vi "灯值调整写入.vi"(8 "error in (no error)":errorcluster, 11 "写入值":cluster{"波长":u16, "ADC":u16, "目标值":u16}={"波长"=365, "ADC"=0, "目标值"=0} {"波长" items=["365"=365, "520"=520, "660"=660]}) -> (0 "error out":errorcluster)   [LabVIEW 2016, in "斯坦道总磷.lvlib"]
uses:
  <vilib>/Plasmionique/MB Master/MB Master.lvlib
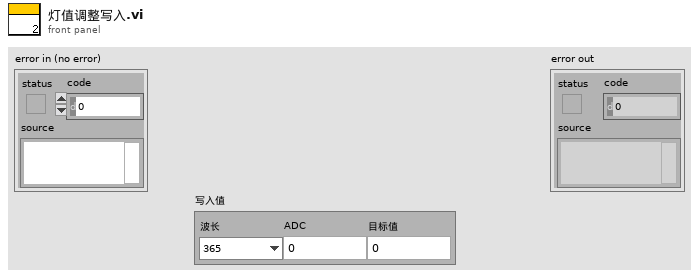
[diagram p1: front panel]
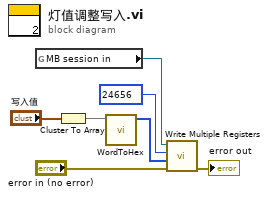
[diagram p0: block diagram]
diagram:
  n1 = global read "VAR总磷总氮全局变量.vi" "MB session in"() -> (w7:refnum<class "MB_Master.lvclass">)
  n2 = Cluster To Array(cluster="写入值") -> (array=w2:u16[])
  n3 = call "WordToHex.vi"("WORD"=w2) -> ("数组"=w1:u16[])  [unwired: 10 in]
  n4 = call <vilib>:"Write Multiple Registers.vi"("error in (no error)"="error in (no error)", "values"=w1, "starting address"=u16 24656, "MB session in"=w7) -> ("error out"=→"error out":errorcluster)  [unwired: 6 in, 1 out]
